vi "Subscriber.vi"() -> ()   [LabVIEW 2019]
uses:
  Parameters.vi
panel:
  in  "stop":bool
  out "Subscriber 1":string
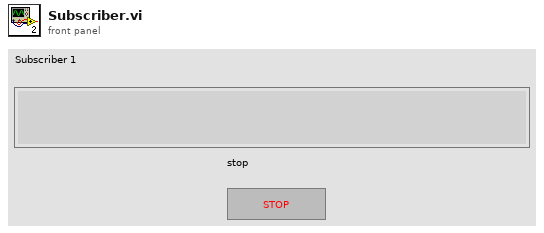
[diagram p1: front panel]
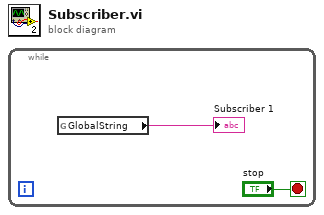
[diagram p0: block diagram]
diagram:
  n1 = while {
    stop <- "stop" stop-if-true
    n2 = global read "Parameters.vi" "GlobalString"() -> (→"Subscriber 1":string)
  }
